vi "Open API Tester.vi"(8 "error in (no error)":errorcluster, 11 "DQMH Library Ref":refnum<vi>) -> (0 "error out":errorcluster)   [LabVIEW 2020, in "Dashboard.lvlib"]
doc: "This VI checks the Main.vi State of the selected DQMH Module"
uses:
  Dashboard.lvlib
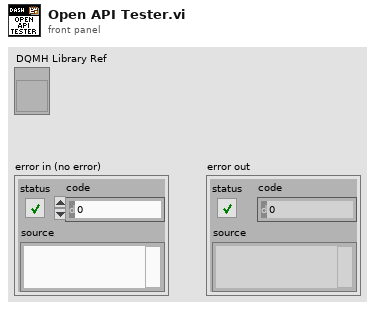
[diagram p1: front panel]
types:
  T1 = enum32{"Bad", "Idle", "Run top level", "Running"}
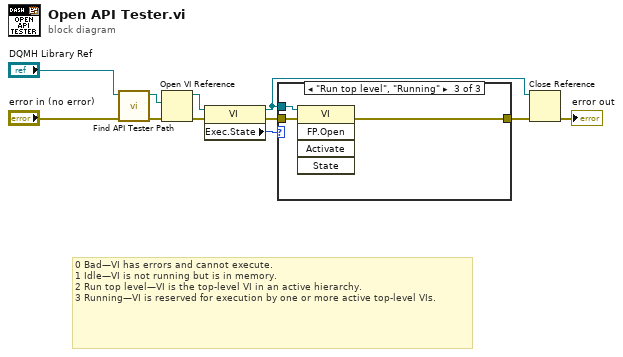
[diagram p0: block diagram]
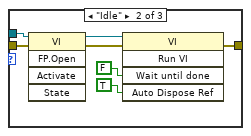
[diagram p3: hidden frame]
diagram:
  # "0\tBad—VI has errors and cannot execute.\n1\tIdle—VI is not running but is in memory.\n2\tRun top level—VI is the top-level VI in an active hierarchy.\n3\tRunning—VI is reserved for execution by one or more active top-level VIs."
  n1 = call "Find API Tester Path.vi"("error in"="error in (no error)", "DQMH Library Ref"="DQMH Library Ref") -> ("error out"=w9:errorcluster, "API Tester Path"=w8:path)  [unwired: 8 in]
  n2 = Open VI Reference(vi path=w8, error in (no error)=w9) -> (vi reference=w6:refnum<vi>, error out=w11:errorcluster)  [unwired: 4 in]
  n3 = property class="VI"(reference=w6, error in=w11) -> (reference out=w1:refnum<vi>, error out=w4:errorcluster, "Exec.State"=w5:T1)
  n4 = case shown="\"Run top level\", \"Running\"" w5 {
    tunnel: w1 -> [_ w15 w21]
    tunnel: w4 -> [w12 w14 w20]
    tunnel: [w12 w13 w22] -> w3
    frame "Bad", Default {
    }
    frame "Idle" {
      n5 = invoke class="VI" method="FP.Open"(reference=w15, error in=w14) -> (reference out=w19:refnum<vi>, error out=w18:errorcluster)  [unwired: 3 in, 3 out]
      n6 = invoke class="VI" method="Run VI"(reference=w19, error in=w18, "Wait until done"=FALSE ("Wait Until Done"), "Auto Dispose Ref"=TRUE ("Auto Dispose Reference")) -> (error out=w13:errorcluster)  [unwired: 1 in, 4 out]
    }
    frame "Run top level", "Running" {
      n7 = invoke class="VI" method="FP.Open"(reference=w21, error in=w20) -> (error out=w22:errorcluster)  [unwired: 3 in, 4 out]
    }
  }
  n8 = Close Reference(reference=w1, error in (no error)=w3) -> (error out=→"error out":errorcluster)
